vi "Write_input_parameters_to_card.vi"(8 "error in (no error)":errorcluster, 10 "Trigger Timeout (10000000)":dbl=1000000.0 min=-1.0 step=1.0, 11 "Control_card in":refnum<class "Control_card.lvclass">) -> (0 "error out":errorcluster, 3 "Control_card out":refnum<class "Control_card.lvclass">)   [LabVIEW 2015, in "Control_card.lvclass"]
uses:
  Control_card.lvclass
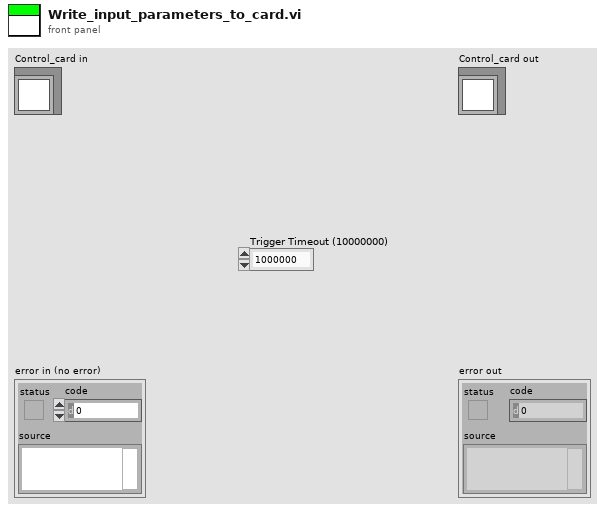
[diagram p1: front panel]
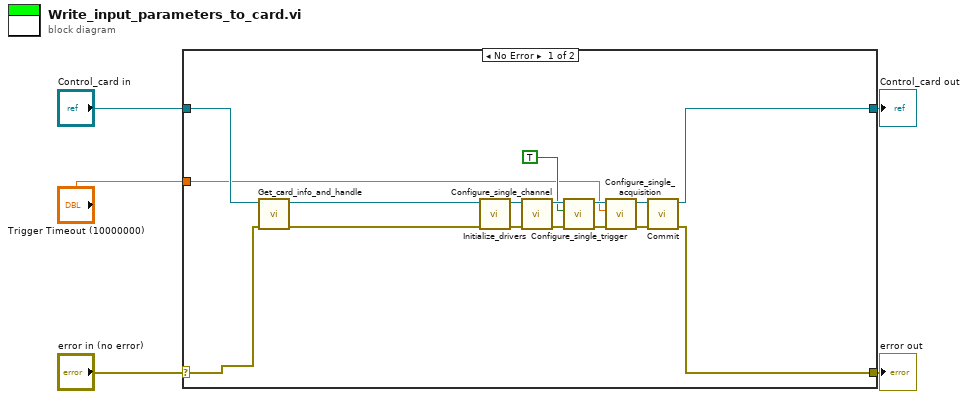
[diagram p0: block diagram]
diagram:
  n1 = case shown="No Error" "error in (no error)" {
    selector: "error in (no error)" -> [w10 w23]
    tunnel: [w8 w22] -> w3
    tunnel: "Control_card in" -> [w16 w22]
    tunnel: [w9 w23] -> w2
    tunnel: "Trigger Timeout (10000000)" -> [w6 _]
    frame No Error {
      n2 = call "Get_card_info_and_handle.vi"("error in (no error)"=w10, "Initialize_card in"=w16) -> ("error out"=w15:errorcluster, "Initialize_card out"=w21:refnum<class "Control_card.lvclass">)  [unwired: 8 in]
      n3 = call-dynamic "Initialize_drivers.vi"("error in (no error)"=w15, "Initialize_card in"=w21) -> ("error out"=w14:errorcluster, "Initialize_card out"=w20:refnum<class "Control_card.lvclass">)  [unwired: 8 in]
      n4 = call-dynamic "Configure_single_channel.vi"("error in (no error)"=w14, "Initialize_card in"=w20) -> ("error out"=w13:errorcluster, "Initialize_card out"=w19:refnum<class "Control_card.lvclass">)  [unwired: 8 in]
      n5 = call-dynamic "Configure_single_trigger.vi"("error in (no error)"=w13, "Enable Trigger?"=TRUE, "Initialize_card in"=w19) -> ("error out"=w12:errorcluster, "Initialize_card out"=w18:refnum<class "Control_card.lvclass">)  [unwired: 7 in]
      n6 = call-dynamic "Configure_single_acquisition.vi"("error in (no error)"=w12, "Trigger Timeout (10000000)"=w6, "Initialize_card in"=w18) -> ("error out"=w11:errorcluster, "Initialize_card out"=w17:refnum<class "Control_card.lvclass">)  [unwired: 7 in]
      n7 = call-dynamic "Commit.vi"("error in (no error)"=w11, "Initialize_card in"=w17) -> ("error out"=w9:errorcluster, "Initialize_card out"=w8:refnum<class "Control_card.lvclass">)  [unwired: 8 in]
    }
    frame Error {
    }
  }
  "error out" <- w2
  "Control_card out" <- w3
